vi "Read-Save Bands.vi"(6 "Task":enum16{"Save", "Read", "List"}(ring)=enum."List", 9 "Name":string="favorites.txt", 11 "Frequencies":dbl[](array[numeric])=[440.0]) -> (0 "file names":string[](array[string]), 1 "String":string, 2 "Long names":string[](array[string]), 3 "Frequencies":dbl[](array[numeric])=[440.0])   [LabVIEW 2022 SP3]
uses:
  <vilib>/Utility/error.llb/Trim Whitespace One-Sided.vi
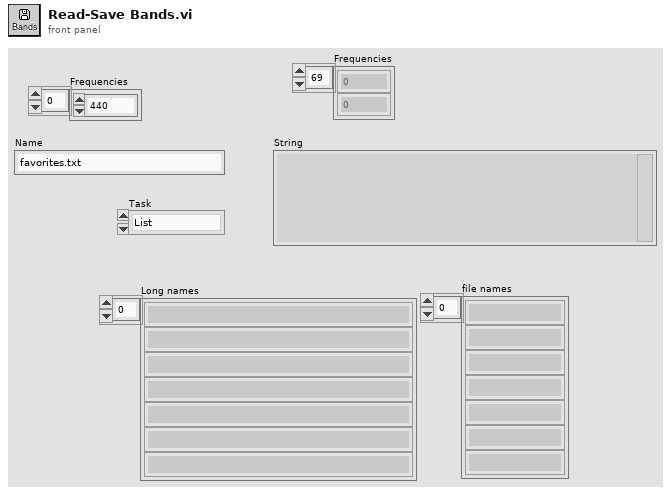
[diagram p1: front panel]
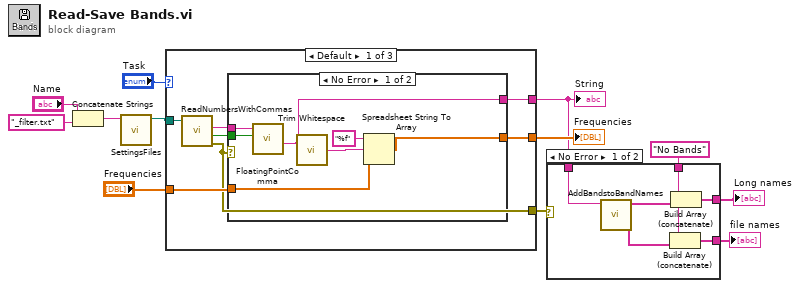
[diagram p0: block diagram]
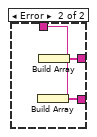
[diagram p2: hidden frame]
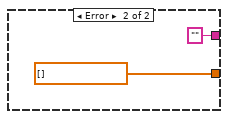
[diagram p3: hidden frame]
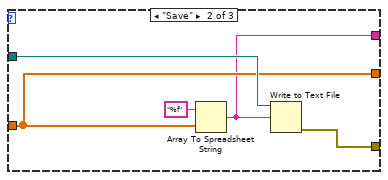
[diagram p4: hidden frame]
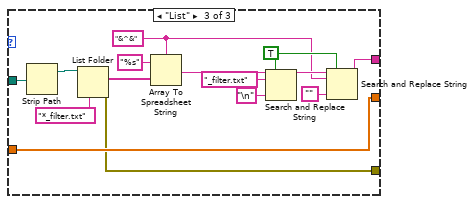
[diagram p5: hidden frame]
diagram:
  n1 = Concatenate Strings("Name", "_filter.txt" ("string")) -> (w1:string)
  n2 = call "SettingsFiles.vi"("settings file name"=w1) -> ("file path"=w2:path)  [unwired: 9 in, 1 out]
  n3 = case shown="Default" "Task" {
    tunnel: "Frequencies" -> [w18 w31 w48]
    tunnel: w2 -> [w16 w33 w47]
    tunnel: [w15 w32 w41] -> w4
    tunnel: [w19 w31 w48] -> w10
    tunnel: [w17 w29 w35] -> w6
    frame Default {
      n4 = call "ReadNumbersWithCommas.vi"("file (use dialog)"=w16) -> ("error out"=w15:errorcluster, "comma?"=w13:bool, "text"=w14:string)  [unwired: 7 in, 1 out]
      n5 = case shown="No Error" w15 {
        tunnel: [w24 dbl[] [] ("DataPath")] -> w19
        tunnel: w14 -> [w22 _]
        tunnel: w18 -> [w26 _]
        tunnel: [w20 ""] -> w17
        tunnel: w13 -> [w21 _]
        frame No Error {
          n6 = call "FloatingPointComma.vi"("Comma?"=w21, "String In"=w22) -> ("fixed"=w20:string)  [unwired: 8 in, 1 out]
          n7 = call <vilib>:"Trim Whitespace.vi"("string"=w20) -> ("trimmed string"=w23:string)  [unwired: 1 in]
          n8 = Spreadsheet String To Array(format string="%f", spreadsheet string=w23, array type (2D Dbl)=w26) -> (array=w24:dbl[])  [unwired: 1 in]
        }
        frame Error {
        }
      }
    }
    frame "Save" {
      n9 = Array To Spreadsheet String(array=w31, 3:"%f" ("format string")) -> (spreadsheet string=w29:string)  [unwired: 1 in]
      n10 = Write to Text File(file (use dialog)=w33, text=w29) -> (error out=w32:errorcluster)  [unwired: 2 in, 2 out]
    }
    frame "List" {
      w34 = "&^&" ("delimiter (Tab)")
      w37 = TRUE ("replace all? (F)")
      n11 = Strip Path(path=w47) -> (stripped path=w46:path)  [unwired: 1 out]
      n12 = List Folder(path=w46, pattern="*_filter.txt") -> (filenames=w44:string[], error out=w41:errorcluster)  [unwired: 2 in, 2 out]
      n13 = Array To Spreadsheet String(delimiter (Tab)=w34, array=w44, 3:"%s" ("format string")) -> (spreadsheet string=w36:string)
      n14 = Search and Replace String(replace all?=w37, input string=w36, search string="_filter.txt", replace string="\n" ("replace string (\"\")")) -> (result string=w38:string)  [unwired: 4 in, 3 out]
      n15 = Search and Replace String(replace all?=w37, input string=w38, search string=w34, replace string="" ("replace string (\"\")")) -> (result string=w35:string)  [unwired: 4 in, 3 out]
    }
  }
  "Frequencies" <- w10
  "String" <- w6
  n16 = case shown="No Error" w4 {
    tunnel: "No Bands" ("String") -> [w50 w55]
    tunnel: w6 -> [w53 _]
    tunnel: [w52 w57] -> w5
    tunnel: [w49 w56] -> w3
    frame No Error {
      n17 = call "AddBandstoBandNames.vi"("filter name"=w53) -> ("File Name"=w51:string[], "Extended Name"=w54:string[])  [unwired: 9 in]
      n18 = Build Array (concatenate)(w50, w51) -> (w49:string[])
      n19 = Build Array (concatenate)(w50, w54) -> (w52:string[])
    }
    frame Error {
      n20 = Build Array(w55) -> (w56:string[])
      n21 = Build Array(w55) -> (w57:string[])
    }
  }
  "Long names" <- w5
  "file names" <- w3
